vi "User_Defined_Test_AdmittanceFilter.vi"() -> (3 "Unit Test Framework Results":T1)   [LabVIEW 2016]
doc: "Use this template to create a user-defined test VI. Define your test requirements and wire the results to the <b>Result (Test)</b> control. Do not modify the <b>Unit Test Framework Results</b> indicator."
uses:
  <vilib>/utf/common/utf_test_result_troll.ctl
  <vilib>/utf/common/utf_test_result.ctl
  <vilib>/utf/common/utf_test_result_failure.ctl
  <vilib>/utf/common/utf_test_comparison_operators.ctl
  <vilib>/utf/common/utf_vi_tag.ctl
  MyPAM Controller/Controls/AdmittanceGains.ctl
  <vilib>/Control Software Solutions Ltd/UTF Helper/SubVIs/UTF Double Equals.vi
  <vilib>/Control Software Solutions Ltd/UTF Helper/SubVIs/UTF Boolean Equals.vi
  MyPAM Controller/controllerLibrary.lvlib
  <vilib>/Control Software Solutions Ltd/UTF Helper/Unit Test Helper.lvlib
  <vilib>/utf/NI_UnitTestFramework.lvlib
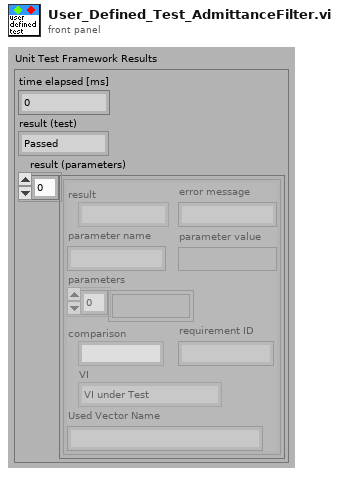
[diagram p1: front panel]
types:
  T1 = typedef "NI_UnitTestFramework.lvlib/utf_test_result_troll.ctl" = cluster{"time elapsed [ms]":u32, "result (test)":T2, "result (parameters)":T3[]}
  T2 = typedef "NI_UnitTestFramework.lvlib/utf_test_result.ctl" = enum16{"Passed", "Failed", "Error", "Skipped", "Not Processed"}
  T3 = typedef "NI_UnitTestFramework.lvlib/utf_test_result_failure.ctl" = cluster{"result":T2, "error message":string, "parameter name":string, "parameter value":variant, "parameters":variant[], "comparison":T4, "requirement ID":string, "VI":T5, "Used Vector Name":string}
  T4 = typedef "NI_UnitTestFramework.lvlib/utf_test_comparison_operators.ctl" = enum16{"=", "!=", ">", ">=", "<", "<=", "range", "symmetric tolerance", "asymmetric tolerance", "string contains", "string not contain", "array size", "string length", "array range", "by element", "array range (limit array)", "user-defined", "array contains", "array not contain", "vector length", "= (elm)", "!= (elm)", "= (case insensitive)", "!= (case insensitive)"}
  T5 = typedef "NI_UnitTestFramework.lvlib/utf_vi_tag.ctl" = enum16{"Setup VI", "VI under Test", "Teardown VI"}
  T6 = typedef "controllerLibrary.lvlib/AdmittanceGains.ctl" = cluster{"C":dbl, "k":dbl}
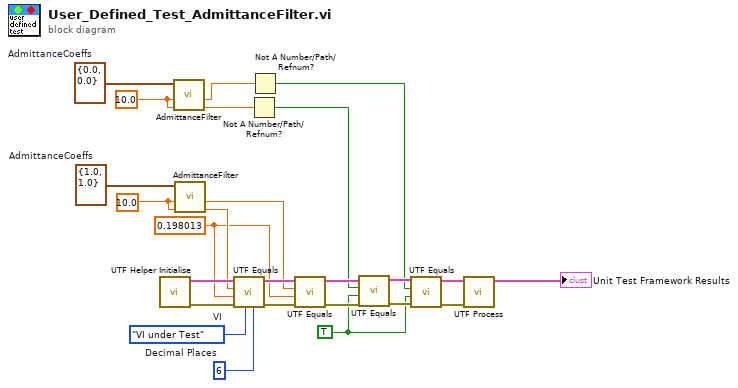
[diagram p0: block diagram]
diagram:
  w3 = TRUE ("Test Value")
  w14 = 10.0 ("Fx")
  w15 = T6 {"C"=0.0, "k"=0.0}  # AdmittanceCoeffs
  w19 = u8 6  # Decimal Places
  w20 = utf_vi_tag."VI under Test"  # VI
  w12 = 0.198013
  w22 = 10.0 ("Fx")
  w23 = T6 {"C"=1.0, "k"=1.0}  # AdmittanceCoeffs
  n1 = call <vilib>:"UTF Helper Initialise.vi"() -> ("error out"=w24:errorcluster, "results array"=w25:T3[])  [unwired: 10 in]
  n2 = call "AdmittanceFilter.vi"("Fy"=w14, "Fx"=w14, "AdmittanceCoeffs"=w15) -> ("Delta y"=w11:dbl, "Delta x"=w2:dbl)  [unwired: 7 in]
  n3 = call "AdmittanceFilter.vi"("Fy"=w22, "Fx"=w22, "AdmittanceCoeffs"=w23) -> ("Delta y"=w21:dbl, "Delta x"=w13:dbl)  [unwired: 7 in]
  n4 = call-poly <vilib>:"UTF Equals.vi"("Decimal Places"=w19, "VI"=w20, "error in (no error)"=w24, "Test Value"=w12, "Input"=w21, "Input Results"=w25) -> ("error out"=w16:errorcluster, "Output Results"=w17:T3[])  [unwired: 4 in]
  n5 = Not A Number/Path/Refnum?(number/path/refnum=w11) -> (NaN/Path/Refnum?=w4:bool)
  n6 = Not A Number/Path/Refnum?(number/path/refnum=w2) -> (NaN/Path/Refnum?=w1:bool)
  n7 = call-poly <vilib>:"UTF Equals.vi"("error in (no error)"=w16, "Test Value"=w12, "Input"=w13, "Input Results"=w17) -> ("error out"=w7:errorcluster, "Output Results"=w8:T3[])  [unwired: 6 in]
  n8 = call-poly <vilib>:"UTF Equals.vi"("error in (no error)"=w7, "Test Value"=w3, "Input"=w4, "Input Results"=w8) -> ("error out"=w6:errorcluster, "Output Results"=w5:T3[])  [unwired: 6 in]
  n9 = call-poly <vilib>:"UTF Equals.vi"("error in (no error)"=w6, "Test Value"=w3, "Input"=w1, "Input Results"=w5) -> ("error out"=w10:errorcluster, "Output Results"=w9:T3[])  [unwired: 6 in]
  n10 = call <vilib>:"UTF Process.vi"("error in (no error)"=w10, "results array"=w9) -> ("Unit Test Framework Results"=→"Unit Test Framework Results":T1)  [unwired: 9 in]
